vi "RegPID.vi"(0 "SP":dbl, 1 "History in":cluster{"I":dbl, "preve":dbl}, 5 "PV":dbl, 7 "Parameters":cluster{"kr":dbl, "TI":dbl, "TD":dbl}, 9 "Limits":cluster{"Upper":dbl, "Lower":dbl}, 12 "h":dbl) -> (3 "History out":cluster{"I":dbl, "preve":dbl}, 4 "CV":dbl, 8 "e":dbl)   [LabVIEW 2017]
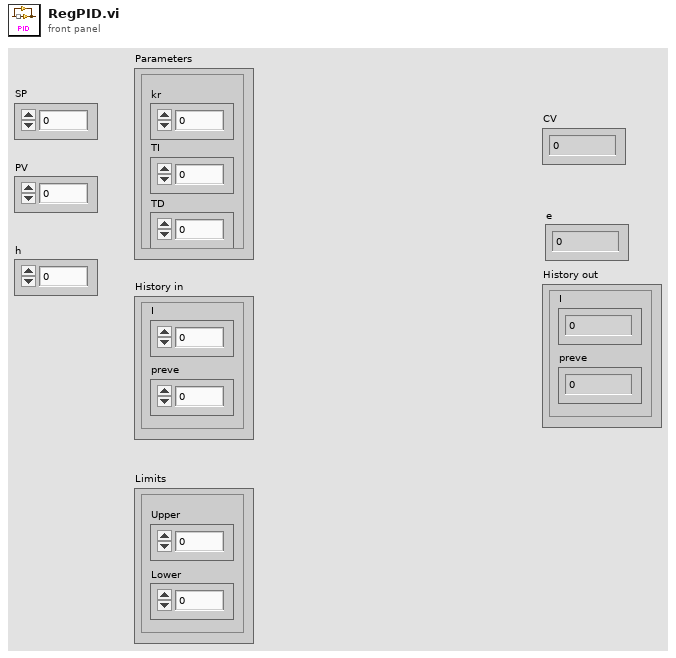
[diagram p1: front panel]
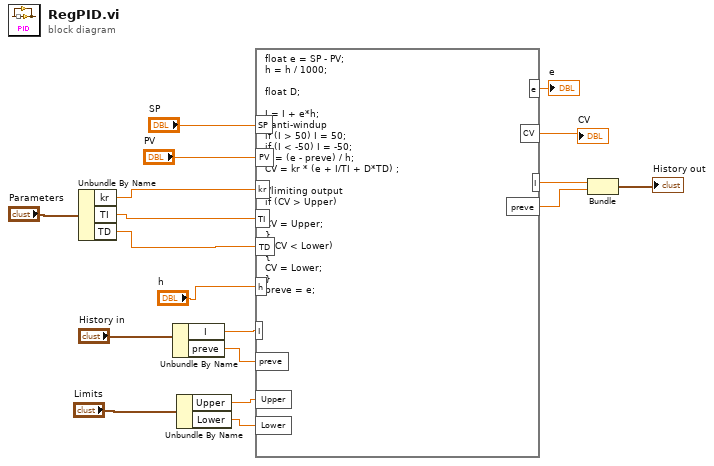
[diagram p0: block diagram]
diagram:
  n1 = Unbundle By Name("Parameters") -> ("kr"=w6:dbl, "TI"=w5:dbl, "TD"=w4:dbl)
  n2 = Unbundle By Name("History in") -> ("I"=w12:dbl, "preve"=w11:dbl)
  n3 = Unbundle By Name("Limits") -> ("Upper"=w2:dbl, "Lower"=w1:dbl)
  n4 = formula code="float e = SP - PV;\nh = h / 1000;\n\nfloat D;\n\nI = I + e*h;\n//anti-windup\nif (I > 50) I = 50;\nif (I < -50) I = -50;\nD = (e - preve) / h;\nCV = kr * (e + I/TI + D*TD) ;\n\n//limiting output\nif (CV > Upper)\n{\nCV = Upper;\n}\nif(CV < Lower)\n{\nCV = Lower;\n}\npreve = e;"("SP"="SP", "PV"="PV", "TI"=w5, "TD"=w4, "kr"=w6, "h"="h", "I"=w12, "preve"=w11, "Upper"=w2, "Lower"=w1) -> ("CV"=→"CV":dbl, "e"=→"e":dbl, "I"=w10:dbl, "preve"=w9:dbl)
  n5 = Bundle("I"=w10, "preve"=w9) -> (→"History out":cluster{"I":dbl, "preve":dbl})  [unwired: 1 in]
